vi "Set Cell Number.vi"(0 "Row":i32, 1 "Col":i32, 2 "Value":dbl format="%.2f", 3 "error in (no error)":errorcluster, 4 "Excel._Worksheet":refnum<k7>) -> (5 "Excel._Worksheet":refnum<k7>, 6 "error out":errorcluster)   [LabVIEW 2012]
doc: "This VI sets the Value of the Cell in the WorkSheet designated by Row:Col to the input \"Value\". It first transforms the numeric row and column inputs to the Excel format of A1, B1 and so on. then it Executes the Range Method of the WorkSheet object and sets the \"Value\" property of the Range. It frees the automation Refnum of Range in each iteration of the loop."
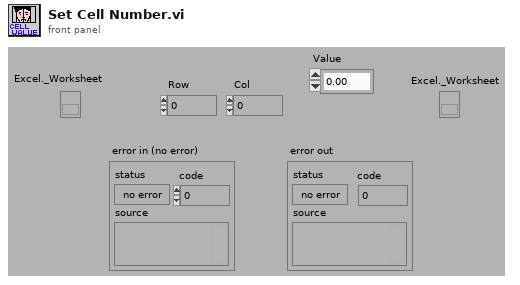
[diagram p1: front panel]
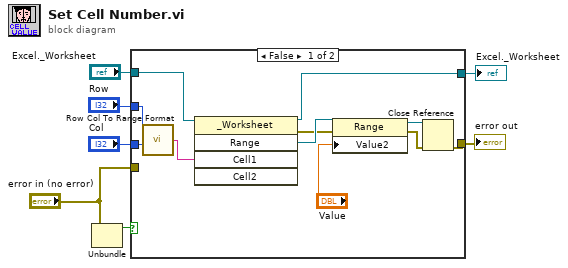
[diagram p0: block diagram]
diagram:
  n1 = Unbundle("error in (no error)") -> ("status"=w3:bool)  [unwired: 2 out]
  n2 = case shown="False" w3 {
    tunnel: "Col" -> [w18 _]
    tunnel: "Row" -> [w17 _]
    tunnel: "error in (no error)" -> [_ w20]
    tunnel: [w10 w20] -> w5
    tunnel: [w9 w19] -> w2
    tunnel: "Excel._Worksheet" -> [w8 w19]
    frame False {
      n3 = call "Row Col To Range Format.vi"("Column"=w18, "Row"=w17) -> ("Output String"=w16:string)
      n4 = invoke class="_Worksheet" method="Range"(reference=w8, "Cell1"=w16) -> (reference out=w9:refnum<k7>, error out=w14:errorcluster, "Range"=w15:refnum<k7>)  [unwired: 3 in, 2 out]
      n5 = property class="Range"(reference=w15, error in=w14, "Value2"="Value") -> (reference out=w12:refnum<k7>, error out=w11:errorcluster)
      n6 = Close Reference(reference=w12, error in (no error)=w11) -> (error out=w10:errorcluster)
    }
    frame True {
    }
  }
  "Excel._Worksheet" <- w2
  "error out" <- w5
